vi "例程04-数组与族.vi"() -> ()   [LabVIEW 2016]
panel:
  out "Boolean 2":bool
  in  "Boolean":bool
  out "Cluster":T1
  out "element":dbl
  out "size(s)":i32[](array[numeric])
  in  "Array":dbl[][](array[numeric])
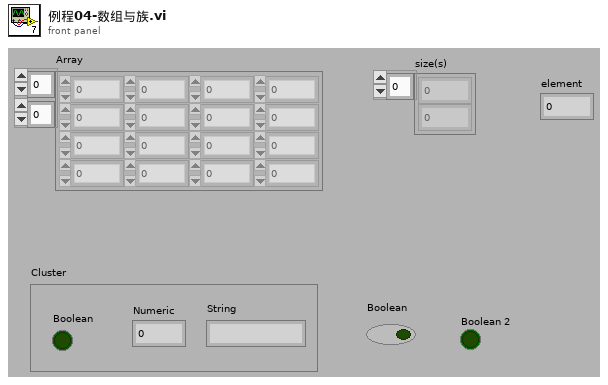
[diagram p1: front panel]
types:
  T1 = cluster{"Boolean":bool, "Numeric":dbl, "String":string}
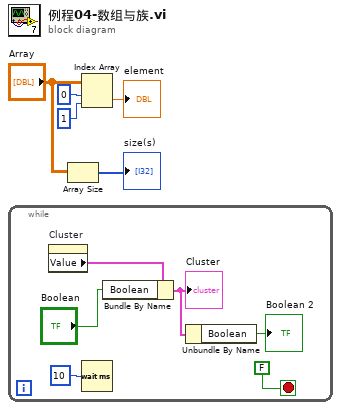
[diagram p0: block diagram]
diagram:
  n1 = while {
    stop <- FALSE stop-if-true
    n2 = property on="Cluster" class="Clust (严格)"() -> ("Value"=w8:T1)  [unwired: 2 in, 2 out]
    n3 = Wait (ms)(milliseconds to wait=u32 10) -> ()  [unwired: 1 out]
    n4 = Bundle By Name(cluster=w8, "Boolean"="Boolean") -> (w7:T1)
    "Cluster" <- w7
    n5 = Unbundle By Name(w7) -> ("Boolean"=→"Boolean 2":bool)
  }
  n6 = Array Size(array="Array") -> (size(s)=→"size(s)":i32[])
  n7 = Index Array(array="Array", index (row)=0, index (col)=1 ("disabled index (col)")) -> (element=→"element":dbl)
